vi "Set Play-Stop buttons.vi"(10 "Function":T1) -> (0 "error out":errorcluster)   [LabVIEW 2013]
uses:
  Typedefs/Select Play-Stop button to show.ctl
  Globals/gl_Time series viewer globals.vi
panel:
  in  "error in (no error)":errorcluster
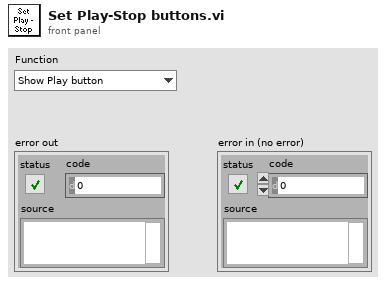
[diagram p1: front panel]
types:
  T1 = typedef "Select Play-Stop button to show.ctl" = enum16{"Show Play button", "Show Stop button"}
  T2 = typedef "Timelapse viewer refs.ctl" = cluster{"This VI":refnum<vi>, "AVI Mode ind":refnum<vi>, "Play":refnum<vi>, "Stop":refnum<vi>, "Back":refnum<vi>, "Scrollbar":refnum<vi>, "Video length info":refnum<vi>, "Expected speed values":refnum<vi>, "Intensity":refnum<vi>, "Path":refnum<vi>, "Selection sliders":refnum<vi>, "Speed Graph ref":refnum<vi>, "Frame rate set (fps)":refnum<vi>}
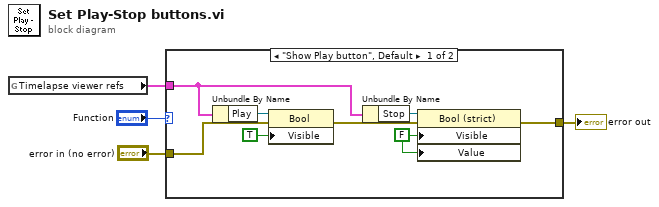
[diagram p0: block diagram]
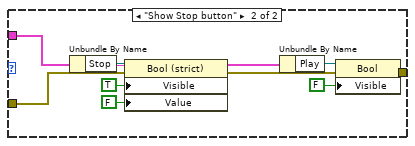
[diagram p2: hidden frame]
diagram:
  n1 = global read "gl_Time series viewer globals.vi" "Timelapse viewer refs"() -> (w3:T2)
  n2 = case shown="\"Show Play button\", Default" "Function" {
    tunnel: [w10 w14] -> w4
    tunnel: w3 -> [w7 w18]
    tunnel: "error in (no error)" -> [w5 w13]
    frame "Show Play button", Default {
      w6 = FALSE ("Visible")
      n3 = Unbundle By Name(w7) -> ("Play"=w11:refnum<vi>)
      n4 = property on="Property Node" class="Bool"(reference=w11, error in=w5, "Visible"=TRUE) -> (error out=w9:errorcluster)  [unwired: 1 out]
      n5 = Unbundle By Name(w7) -> ("Stop"=w12:refnum<vi>)
      n6 = property on="Property Node" class="Bool (strict)"(reference=w12, error in=w9, "Visible"=w6, "Value"=w6) -> (error out=w10:errorcluster)  [unwired: 1 out]
    }
    frame "Show Stop button" {
      n7 = Unbundle By Name(w18) -> ("Stop"=w21:refnum<vi>)
      n8 = property on="Property Node" class="Bool (strict)"(reference=w21, error in=w13, "Visible"=TRUE, "Value"=FALSE) -> (error out=w15:errorcluster)  [unwired: 1 out]
      n9 = Unbundle By Name(w18) -> ("Play"=w20:refnum<vi>)
      n10 = property on="Property Node" class="Bool"(reference=w20, error in=w15, "Visible"=FALSE) -> (error out=w14:errorcluster)  [unwired: 1 out]
    }
  }
  "error out" <- w4
